vi "To String.vi"(8 "error in (no error)":errorcluster, 11 "Cluster Array in":refnum<class "Cluster Array.lvclass">) -> (0 "error out":errorcluster, 2 "String":string)   [LabVIEW 2020, in "Data.lvlib" / "Cluster Array.lvclass"]
doc: "Convert 'Generic Data in' to a string."
uses:
  Cluster Array.lvclass
  Cluster Array.lvclass/Cluster Array.ctl
  Cluster/Cluster.lvclass
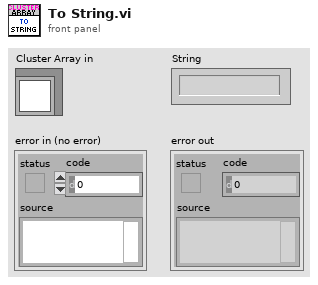
[diagram p1: front panel]
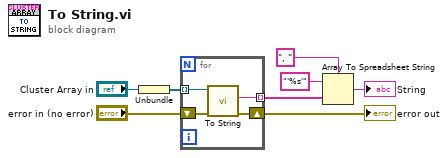
[diagram p0: block diagram]
diagram:
  n1 = Unbundle("Cluster Array in") -> (w4:refnum<class "Cluster.lvclass">[])
  n2 = for {
    tunnel: w4 -> [w12] mode=indexing
    tunnel: [w11] -> w3 mode=indexing
    shift-right: [w9] -> w1
    shift-left: "error in (no error)" -> [w10]
    n3 = call-dynamic "To String.vi"("error in (no error)"=w10, "Cluster in"=w12) -> ("error out"=w9:errorcluster, "String"=w11:string)  [unwired: 8 in]
  }
  "error out" <- w1
  n4 = Array To Spreadsheet String(delimiter (Tab)=", ", array=w3, 3:"'%s'" ("format string")) -> (spreadsheet string=→"String":string)
